vi "Add.vi"(8 "error in (no error)":errorcluster, 10 "High Res Arithmetic 2":refnum<class "High Res Arithmetic.lvclass">, 11 "High Res Arithmetic 1":refnum<class "High Res Arithmetic.lvclass">) -> (0 "error out":errorcluster, 3 "High Res Arithmetic sum":refnum<class "High Res Arithmetic.lvclass">)   [LabVIEW 2021, in "High Res Arithmetic.lvclass"]
uses:
  High Res Arithmetic.lvclass
  High Res Arithmetic.lvclass/High Res Arithmetic.ctl
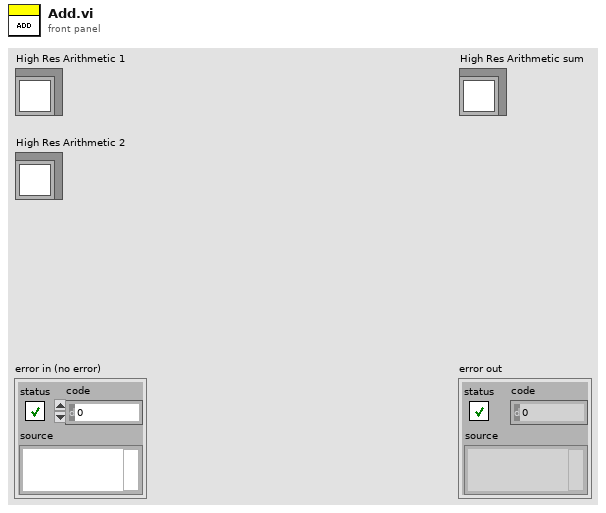
[diagram p1: front panel]
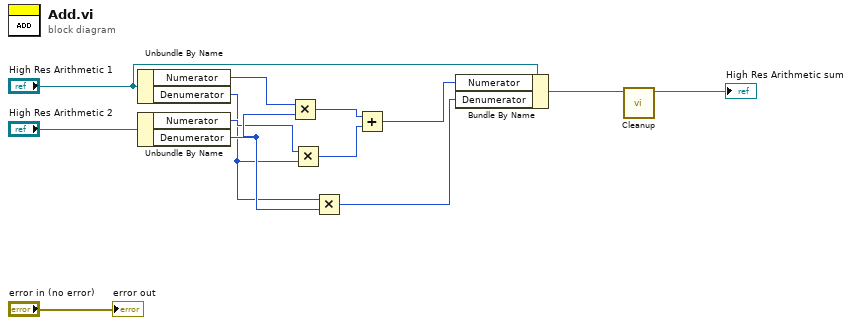
[diagram p0: block diagram]
diagram:
  n1 = Unbundle By Name("High Res Arithmetic 1") -> ("Numerator"=w10:i64, "Denumerator"=w7:i64)
  n2 = Unbundle By Name("High Res Arithmetic 2") -> ("Numerator"=w8:i64, "Denumerator"=w9:i64)
  n3 = Multiply(x=w10, y=w9) -> (x*y=w6:i64)
  n4 = Multiply(x=w8, y=w7) -> (x*y=w5:i64)
  n5 = Multiply(x=w7, y=w9) -> (x*y=w3:i64)
  n6 = Add(x=w6, y=w5) -> (x+y=w4:i64)
  n7 = Bundle By Name(cluster="High Res Arithmetic 1", "Numerator"=w4, "Denumerator"=w3) -> (w2:refnum<class "High Res Arithmetic.lvclass">)
  n8 = call "Cleanup.vi"("High Res Arithmetic in"=w2) -> ("High Res Arithmetic out"=→"High Res Arithmetic sum":refnum<class "High Res Arithmetic.lvclass">)  [unwired: 9 in, 1 out]
  "error out" <- "error in (no error)"
